vi "RSZVB Get Virtual Transform Ground Loop State.vi"(8 "error in (no error)":errorcluster {"code" format="%.0x"}, 9 "Function Type (0)":i32(ring) items=["Deembedding", "Embedding"], 10 "Channel (1)":i32=1, 11 "VISA session":refnum<visa-resource-name>) -> (0 "error out":errorcluster {"code" format="%.0x"}, 1 "State":bool, 3 "dup VISA session":refnum<visa-resource-name>)   [LabVIEW 2011]
doc: "This VI returns the state of the deembedding/embedding VI for ground loops. It is allowed to change the circuit model and its parameters while deembedding is enabled.\n\nRemote-control command(s):\nCALCulate<Ch>:TRANsform:VNETworks:GLOop:DEEMbedding[:STATe]?\nCALCulate<Ch>:TRANsform:VNETworks:GLOop:EMBedding[:STATe]?"
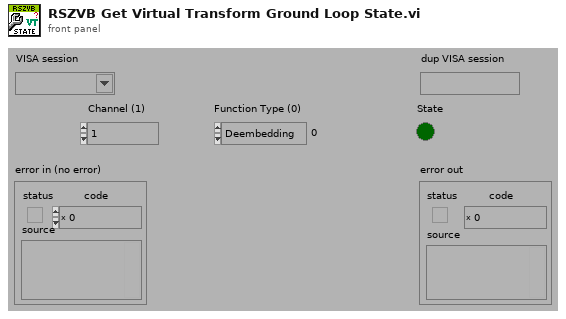
[diagram p1: front panel]
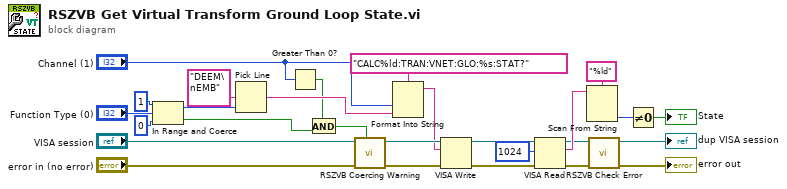
[diagram p0: block diagram]
diagram:
  n1 = In Range and Coerce(upper limit=1, x="Function Type (0)", lower limit=0) -> (coerced(x)=w22:i32, In Range?=w19:bool)
  n2 = Pick Line(multi-line string="DEEM\nEMB", line index=w22) -> (output string=w18:string)  [unwired: 1 in]
  n3 = Greater Than 0?(x="Channel (1)") -> (x > 0?=w17:bool)
  n4 = And(x=w17, y=w19) -> (x .and. y?=w16:bool)
  n5 = call "RSZVB Coercing Warning.vi"("In Range?"=w16, "error in (no error)"="error in (no error)", "VISA session"="VISA session") -> ("error out"=w25:errorcluster, "dup VISA session"=w26:refnum<visa-resource-name>)  [unwired: 7 in]
  n6 = Format Into String(format string="CALC%ld:TRAN:VNET:GLO:%s:STAT?", "Channel (1)", w18) -> (resulting string=w24:string)  [unwired: 2 in, 1 out]
  n7 = VISA Write(VISA resource name=w26, write buffer=w24, error in (no error)=w25) -> (VISA resource name out=w7:refnum<visa-resource-name>, error out=w6:errorcluster)  [unwired: 1 out]
  n8 = VISA Read(VISA resource name=w7, byte count=u32 1024 ("byte count (0)"), error in (no error)=w6) -> (VISA resource name out=w9:refnum<visa-resource-name>, read buffer=w11:string, error out=w10:errorcluster)  [unwired: 1 out]
  n9 = Scan From String(format string="%ld", input string=w11) -> (output 1=w4:i32)  [unwired: 3 in, 3 out]
  n10 = call "RSZVB Check Error.vi"("error in (no error)"=w10, "VISA session"=w9) -> ("error out"=→"error out":errorcluster, "dup VISA session"=→"dup VISA session":refnum<visa-resource-name>)  [unwired: 8 in]
  n11 = Not Equal To 0?(x=w4) -> (x != 0?=→"State":bool)
